vi "Write NumberOfRobots.vi"(8 "error in (no error)":errorcluster, 10 "NumberOfRobots":dbl, 11 "DirectEnemyPlay in":refnum<class "DirectEnemyPlay.lvclass">) -> (0 "error out":errorcluster, 3 "DirectEnemyPlay out":refnum<class "DirectEnemyPlay.lvclass">)   [LabVIEW 2020, in "DirectEnemyPlay.lvclass"]
uses:
  DirectEnemyPlay.lvclass
  DirectEnemyPlay.lvclass/DirectEnemyPlay.ctl
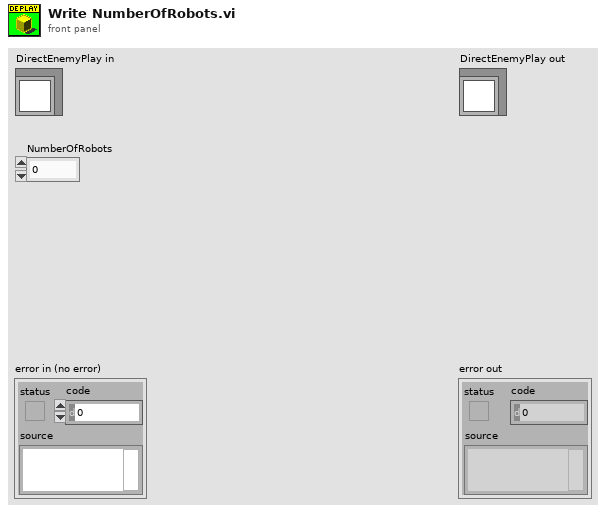
[diagram p1: front panel]
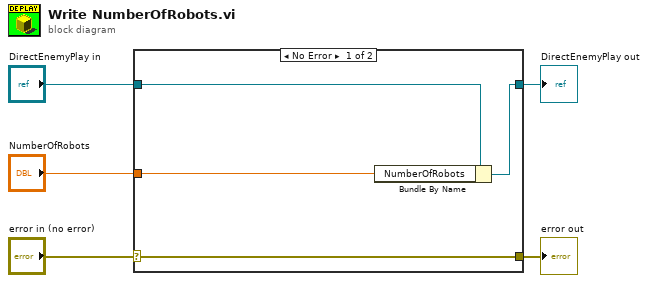
[diagram p0: block diagram]
diagram:
  n1 = case shown="No Error" "error in (no error)" {
    selector: "error in (no error)" -> [w9 w10]
    tunnel: [w9 w10] -> w4
    tunnel: [w7 w11] -> w2
    tunnel: "DirectEnemyPlay in" -> [w8 w11]
    tunnel: "NumberOfRobots" -> [w6 _]
    frame No Error {
      n2 = Bundle By Name(cluster=w8, "NumberOfRobots"=w6) -> (w7:refnum<class "DirectEnemyPlay.lvclass">)
    }
    frame Error {
    }
  }
  "error out" <- w4
  "DirectEnemyPlay out" <- w2
